vi "New HTS221.vi"(8 "error in (no error)":errorcluster, 11 "I2C in":refnum<class "LINX I2C.lvclass">) -> (0 "error out":errorcluster, 3 "HTS221 out":refnum<class "HTS221.lvclass">)   [LabVIEW 2020, in "HTS221.lvclass"]
doc: "Creates a new HTS221 object from the I2C configuration."
uses:
  HTS221.lvclass
  LINX I2C/LINX I2C.lvclass
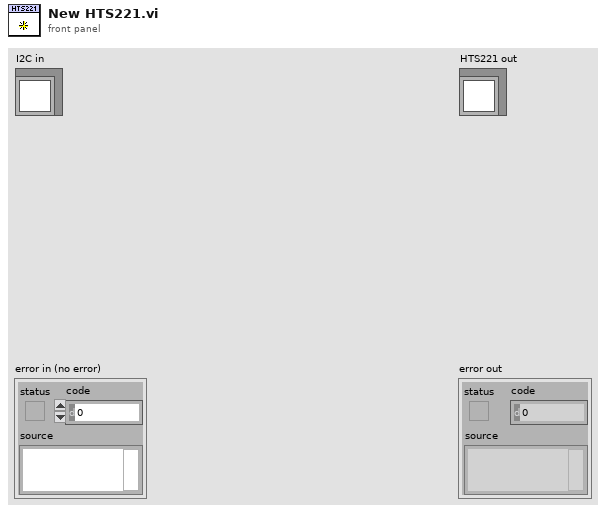
[diagram p1: front panel]
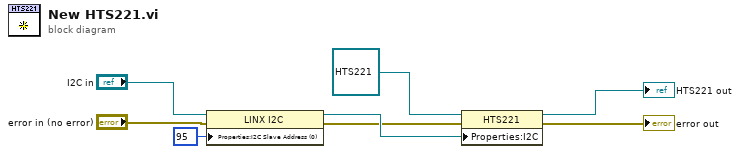
[diagram p0: block diagram]
diagram:
  n1 = property class="LINX I2C"(reference="I2C in", error in="error in (no error)", "Properties:I2C Slave Address (0)"=u8 95 ("I2C Slave Address (0)")) -> (reference out=w5:refnum<class "LINX I2C.lvclass">, error out=w4:errorcluster)
  n2 = property class="HTS221"(reference=refnum<class "HTS221.lvclass"> refnum ("HTS221 out"), error in=w4, "Properties:I2C"=w5) -> (reference out=→"HTS221 out":refnum<class "HTS221.lvclass">, error out=→"error out":errorcluster)
